vi "AIDI-Configure AI.vi"(0 "AI.Channels":string[](array[string]), 5 "AI.Fs (Hz)":dbl, 7 "AI.Npts":i32, 11 "error in (no error)":errorcluster) -> (15 "error out":errorcluster)   [LabVIEW 2020]
uses:
  Typedefs/AIDI-Config.ctl
  Typedefs/AIDI-Output Spec.ctl
  Typedefs/DI-Output Spec.ctl
  Typedefs/AIDI-Action.ctl
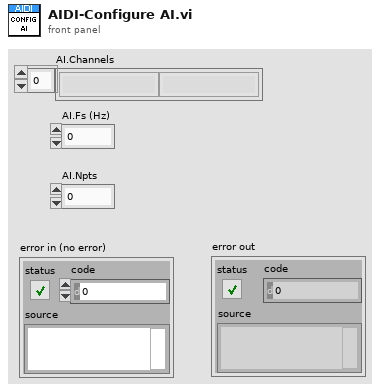
[diagram p1: front panel]
types:
  T1 = typedef "AIDI-Action.ctl" = enum16{"Configure", "Initialize", "Start", "Read", "Clean up", "Init & Start", "Config & Test", "Position"}
  T2 = typedef "AIDI-Config.ctl" = cluster{"AI":T3, "DI":T4, "ExtTrig":bool}
  T3 = typedef "AIDI-Output Spec.ctl" = cluster{"Channels":string[], "Fs (Hz)":dbl, "Npts":i32}
  T4 = typedef "DI-Output Spec.ctl" = cluster{"Channels":string[], "Fs (Hz)":dbl, "Npts":i32, "Port":string}
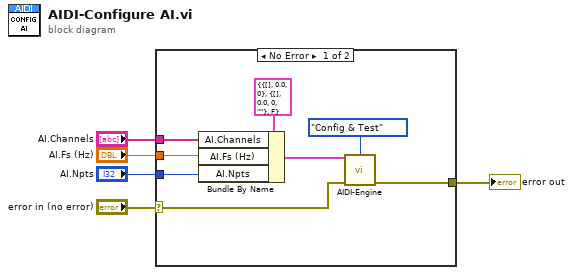
[diagram p0: block diagram]
diagram:
  n1 = case shown="No Error" "error in (no error)" {
    selector: "error in (no error)" -> [w7 w14]
    tunnel: "AI.Channels" -> [w10 _]
    tunnel: "AI.Fs (Hz)" -> [w9 _]
    tunnel: "AI.Npts" -> [w8 _]
    tunnel: [w6 w14] -> w1
    frame No Error {
      n2 = Bundle By Name(cluster=T2 {"AI"={"Channels"=[], "Fs (Hz)"=0.0, "Npts"=0}, "DI"={"Channels"=[], "Fs (Hz)"=0.0, "Npts"=0, "Port"=""}, "ExtTrig"=FALSE} ("Config"), "AI.Channels"=w10, "AI.Fs (Hz)"=w9, "AI.Npts"=w8) -> (w12:T2)
      n3 = call "AIDI-Engine.vi"("Config"=w12, "Action"=AIDI-Action."Config & Test", "error in (no error)"=w7) -> ("error out"=w6:errorcluster)  [unwired: 9 in, 3 out]
    }
    frame Error {
    }
  }
  "error out" <- w1
